vi "SetAttributeViString_SA-HD_OB.vi"(7 "AttributeValue":string, 8 "error in (no error)":errorcluster {"code" format="%.0x"}, 9 "AttributeID":u32(ring)=1150311 items=["SA_OCCUPIEDBANDWIDTH_DISPLAY_TEXT"=1150311], 11 "instrument handle":refnum<k15>) -> (0 "error out":errorcluster {"code" format="%.0x"}, 3 "instrument handle out":refnum<k15>)   [LabVIEW 2009, in "Keysight XSAn.lvlib"]
doc: "Sets a String attribute from the instrument driver.\nThe following Attributes are supported:\n\nSA_OCCUPIEDBANDWIDTH_DISPLAY_TEXT"
uses:
  <instrlib>/Keysight XSAn/Keysight XSAn.lvlib
  AgXSAn.dll
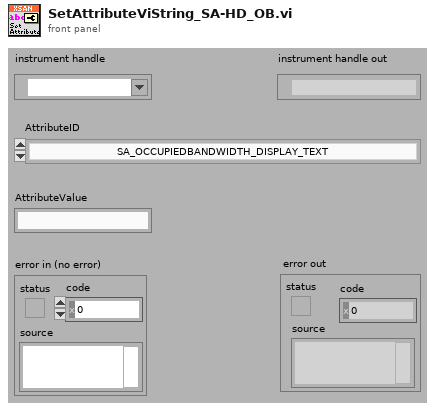
[diagram p1: front panel]
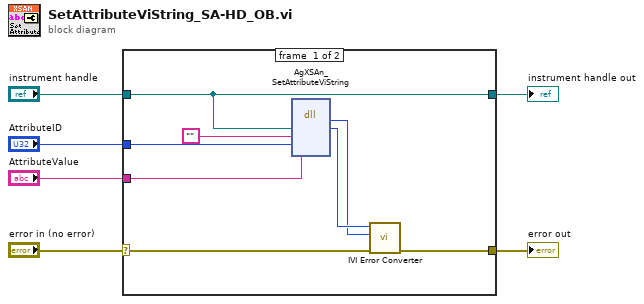
[diagram p0: block diagram]
diagram:
  n1 = case shown="No Error" "error in (no error)" {
    selector: "error in (no error)" -> [w12 w16]
    tunnel: [w11 w16] -> w6
    tunnel: "instrument handle" -> [w8 w15]
    tunnel: "AttributeID" -> [w10 _]
    tunnel: "AttributeValue" -> [w9 _]
    tunnel: [w8 w15] -> w1
    frame #0 {
      n2 = dll-call lib="AgXSAn**.dll" fn="AgXSAn_SetAttributeViString"("Vi"=w8, "RepCapIdentifier"="", "AttributeID"=w10, "AttributeValue"=w9) -> ("return type"=w13:i32, "Vi"=w14:u32)  [unwired: 6 in, 2 out]
      n3 = call <instrlib>:"IVI Error Converter.vi"("error in (no error)"=w12, "IVI error code (0)"=w13, "instrument handle"=w14) -> ("error out"=w11:errorcluster)  [unwired: 7 in, 1 out]
    }
    frame #1 {
    }
  }
  "error out" <- w6
  "instrument handle out" <- w1
